vi "_Select Single.vi"(0 "Socket":u32 format="%x", 1 "Mode (Read)":enum16{"Read", "Write", "Errors"}(ring), 11 "Error In":errorcluster, 12 "Timeout (ms)":i32) -> (4 "Socket Out":u32 format="%x", 6 "Timeout?":bool, 8 "Socket Ready?":bool, 14 "RxTimeStamp":u32, 15 "Error Out":errorcluster)   [LabVIEW 2018]
uses:
  ws2_32.dll
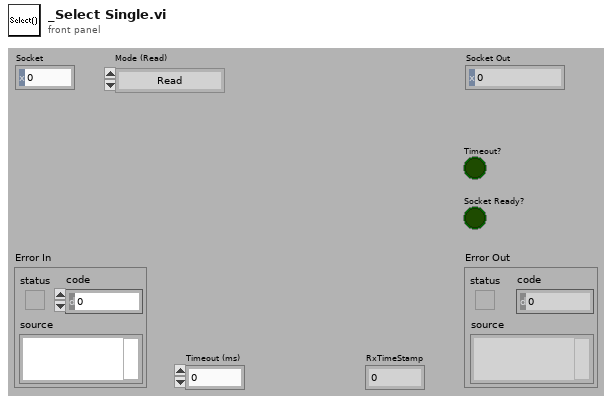
[diagram p1: front panel]
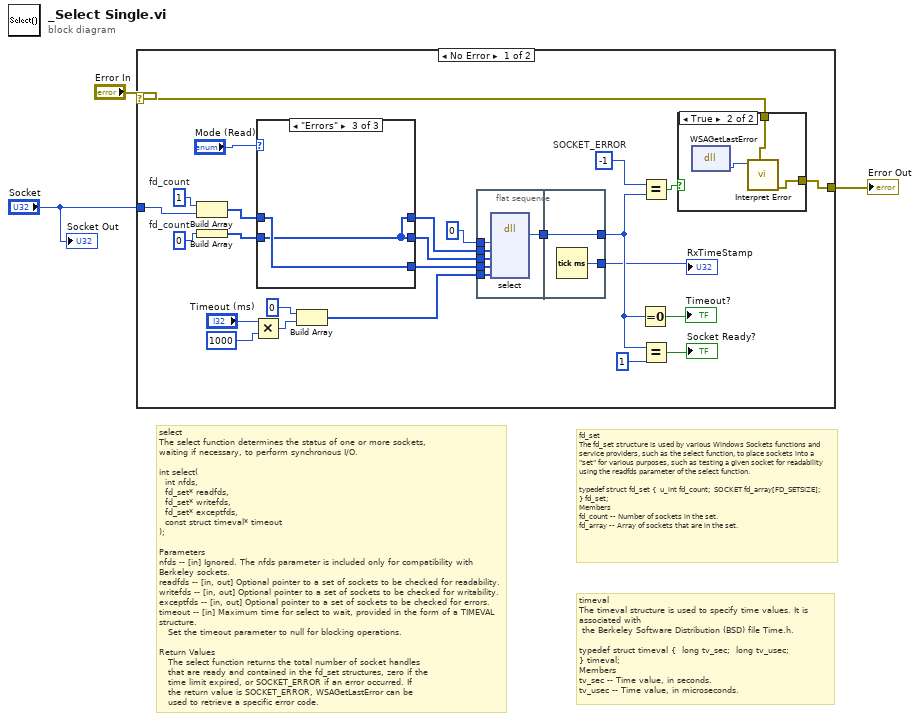
[diagram p0: block diagram]
diagram:
  # "timeval\nThe timeval structure is used to specify time values. It is associated with\n the Berkeley Software Distribution (BSD) file Time.h.\n\ntypedef struct timeval {  long tv_sec;  long tv_usec;\n} timeval;\nMembers\ntv_sec -- Time value, in seconds. \ntv_usec -- Time value, in microseconds."
  # "fd_set\nThe fd_set structure is used by various Windows Sockets functions and \nservice providers, such as the select function, to place sockets into a \n\"set\" for various purposes, such as testing a given socket for readability \nusing the readfds parameter of the select function.\n\ntypedef struct fd_set {  u_int fd_count;  SOCKET fd_array[FD_SETSIZE];\n} fd_set;\nMembers\nfd_count -- Number of sockets in the set. \nfd_array -- Array of sockets that are in the set."
  # "select\nThe select function determines the status of one or more sockets, \nwaiting if necessary, to perform synchronous I/O.\n\nint select(\n  int nfds,\n  fd_set* readfds,\n  fd_set* writefds,\n  fd_set* exceptfds,\n  const struct timeval* timeout\n);\n\nParameters\nnfds -- [in] Ignored. The nfds parameter is included only for compatibility with Berkeley sockets. \nreadfds -- [in, out] Optional pointer to a set of sockets to be checked for readability. \nwritefds -- [in, out] Optional pointer to a set of sockets to be checked for writability. \nexceptfds -- [in, out] Optional pointer to a set of sockets to be checked for errors. \ntimeout -- [in] Maximum time for select to wait, provided in the form of a TIMEVAL structure. \n   Set the timeout parameter to null for blocking operations. \n\nReturn Values\n   The select function returns the total number of socket handles \n   that are ready and contained in the fd_set structures, zero if the \n   time limit expired, or SOCKET_ERROR if an error occurred. If \n   the return value is SOCKET_ERROR, WSAGetLastError can be \n   used to retrieve a specific error code."
  n1 = case shown="No Error" "Error In" {
    selector: "Error In" -> [w28 w47]
    tunnel: [w27 w47] -> w2
    tunnel: "Socket" -> [w21 _]
    frame No Error {
      w7 = u32 0  # fd_count
      w8 = u32 1  # fd_count
      w11 = -1  # SOCKET_ERROR
      n2 = Build Array(w8, w21) -> (w19:u32[])
      n3 = Build Array(w7) -> (w6:u32[])
      n4 = Multiply(x="Timeout (ms)", y=1000) -> (x*y=w24:i32)
      n5 = case shown="\"Errors\"" "Mode (Read)" {
        tunnel: w19 -> [w38 w40 w42]
        tunnel: [w38 w39 w41] -> w18
        tunnel: [w37 w40 w41] -> w17
        tunnel: [w37 w39 w42] -> w16
        tunnel: w6 -> [w37 w39 w41]
        frame "Read", Default {
        }
        frame "Write" {
        }
        frame "Errors" {
        }
      }
      n6 = Build Array(0 ("element"), w24) -> (w22:i32[])
      n7 = flat-sequence {
        tunnel: w22 -> [w34]
        tunnel: w18 -> [w33]
        tunnel: w17 -> [w32]
        tunnel: w16 -> [w31]
        tunnel: 0 ("nfds") -> [w29]
        tunnel: [w30] -> w5
        tunnel: [w36] -> w14
        tunnel: w5 -> [w36]
        tunnel: [w35] -> w4
        frame #0 {
          n8 = dll-call lib="ws2_32.dll" fn="select" label="Select()"("nfds"=w29, "readfds"=w33, "writefds"=w32, "exceptfds"=w31, "Timeout"=w34) -> (w30:i32)  [unwired: 8 in, 2 out]
        }
        frame #1 {
          n9 = Tick Count (ms)() -> (millisecond timer value=w35:u32)
        }
      }
      n10 = Equal To 0?(x=w14) -> (x = 0?=→"Timeout?":bool)
      n11 = Equal?(x=w11, y=w14) -> (x = y?=w26:bool)
      n12 = Equal?(x=w14, y=1) -> (x = y?=→"Socket Ready?":bool)
      n13 = case shown="True" w26 {
        tunnel: w28 -> [w43 w45]
        tunnel: [w43 w44] -> w27
        frame False {
        }
        frame True {
          n14 = dll-call lib="ws2_32.dll" fn="WSAGetLastError"() -> (w46:i32)  [unwired: 3 in, 2 out]
          n15 = call "Interpret Error.vi"("Error In"=w45, "Code"=w46) -> ("Error Out"=w44:errorcluster)  [unwired: 9 in]
        }
      }
      "RxTimeStamp" <- w4
    }
    frame Error {
    }
  }
  "Error Out" <- w2
  "Socket Out" <- "Socket"
